vi "STD电导率_获取温度和测量值.vi"(8 "error in (no error)":errorcluster caption="错误输入（无错误）", 11 "MB session in":refnum<class "MB_Master.lvclass">) -> (0 "error out":errorcluster caption="错误输出", 2 "STDspcond":cluster{"温度测量值":sgl, "测量值":sgl, "信号值":sgl}, 3 "MB session out":refnum<class "MB_Master.lvclass">)   [LabVIEW 2016, in "斯坦道多参数.lvlib"]
uses:
  <vilib>/Plasmionique/MB Master/MB_Master/MB_Master.lvclass
  <vilib>/Plasmionique/MB Master/MB Master.lvlib
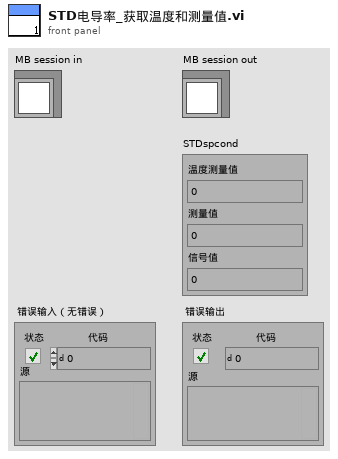
[diagram p1: front panel]
types:
  T1 = cluster{"pH":u32, "DO":u32, "Cond":u32, "Turb":u32, "叶绿素a":u32, "藻密度":u32, "ORP":u32, "COD":u32, "氯化物":u32, "氨氮":u32, "水中油":u32, "悬浮物":u32, "余氯":u32}
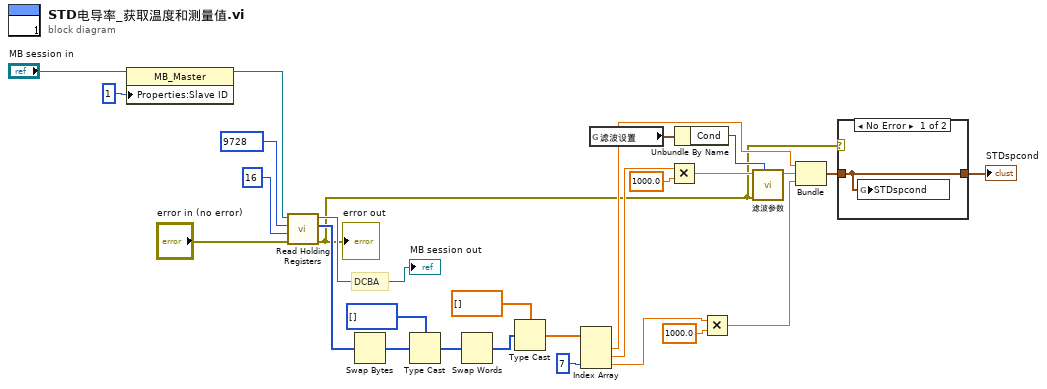
[diagram p0: block diagram]
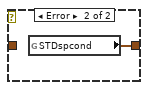
[diagram p2: hidden frame]
diagram:
  # "DCBA"
  n1 = property class="MB_Master"(reference="MB session in", "Properties:Slave ID"=u16 1 ("y")) -> (reference out=w20:refnum<class "MB_Master.lvclass">)  [unwired: 1 in, 1 out]
  n2 = call <vilib>:"Read Holding Registers.vi"("error in (no error)"="error in (no error)", "quantity"=u16 16, "starting address"=u16 9728, "MB session in"=w20) -> ("error out"=w7:errorcluster, "Registers"=w18:u16[], "MB session out"=→"MB session out":refnum<class "MB_Master.lvclass">)  [unwired: 5 in]
  "error out" <- w7
  n3 = Swap Bytes(anything=w18) -> (byte swapped=w4:u16[])
  n4 = Type Cast(type=u32[] [] ("数组 2"), x=w4) -> (*(type *) &x=w24:u32[])
  n5 = Swap Words(1:w24) -> (0:w26:u32[])
  n6 = Type Cast(type=sgl[] [] ("数组 2"), x=w26) -> (*(type *) &x=w22:sgl[])
  n7 = Index Array(array=w22, index #3=7 ("索引")) -> (element #1=w17:sgl, element #2=w16:sgl, element #3=w1:sgl)  [unwired: 2 in]
  n8 = global read "断电保存变量.vi" "滤波设置"() -> (w9:T1)
  n9 = Multiply(x=w16, y=sgl 1000.0) -> (x*y=w11:sgl)
  n10 = Unbundle By Name(w9) -> ("Cond"=w8:u32)
  n11 = Multiply(x=w1, y=sgl 1000.0) -> (x*y=w2:sgl)
  n12 = call "滤波参数.vi"("滤波次数"=w8, "error in (no error)"=w7, "x"=w11) -> ("mode"=w10:dbl)  [unwired: 7 in, 1 out]
  n13 = Bundle("数值"=w17, "mode"=w10, w2) -> (w14:cluster{"数值":sgl, "mode":dbl, sgl})  [unwired: 1 in]
  n14 = case shown="No Error" w7 {
    tunnel: w14 -> [w29 _]
    tunnel: [w29 w30] -> w6
    frame No Error {
      n15 = global write "禹山过程全局变量.vi" "STDspcond"(w29) -> ()
    }
    frame Error {
      n16 = global read "禹山过程全局变量.vi" "STDspcond"() -> (w30:cluster{"温度测量值":sgl, "测量值":sgl, "信号值":sgl})
    }
  }
  "STDspcond" <- w6
